vi "Get StationGlobal.vi"() -> ()   [LabVIEW 2019]
uses:
  Engine/Engine.lvclass
  VariableContainer/VariableContainer.lvclass
panel:
  out "error out":errorcluster
  out "Original Value":string="UnlikelyNomad"
  in  "Lookup String":string="Channel"
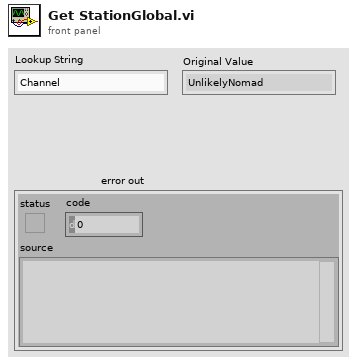
[diagram p1: front panel]
types:
  T1 = typedef "HTS.lvlib/Engine.lvclass/Session Handle.ctl" = refnum<data-value>
  T2 = typedef "HTS.lvlib/VariableContainer.lvclass/Session Handle.ctl" = refnum<data-value>
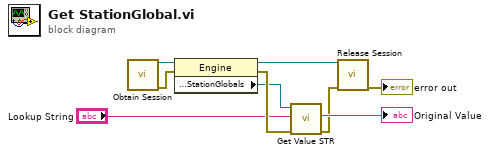
[diagram p0: block diagram]
diagram:
  n1 = call "Obtain Session.vi"() -> ("Session Handle"=w6:T1, "error out"=w8:errorcluster)  [unwired: 14 in]
  n2 = property class="Engine"(reference=w6, error in=w8) -> (reference out=w5:T1, error out=w7:errorcluster, "Properties:StationGlobals"=w4:T2)
  n3 = call "Get Value STR.vi"("error in (no error)"=w7, "Lookup String"="Lookup String", "Session Handle in"=w4) -> ("error out"=w2:errorcluster, "Value"=→"Original Value":string)  [unwired: 6 in, 1 out]
  n4 = call "Release Session.vi"("Session Handle"=w5, "error in (no error)"=w2) -> ("error out"=→"error out":errorcluster)  [unwired: 13 in]
